vi "Destroy StateMachine.vi"(8 "error in (no error)":errorcluster, 11 "statemachine in":refnum<class "statemachine.lvclass">) -> (0 "error out":errorcluster, 3 "statemachine out":refnum<class "statemachine.lvclass">)   [LabVIEW 2020, in "eos.lvlib" / "statemachine.lvclass"]
uses:
  statemachine.lvclass
  statemachine.lvclass/statemachine.ctl
  interfaces/data/data.lvclass
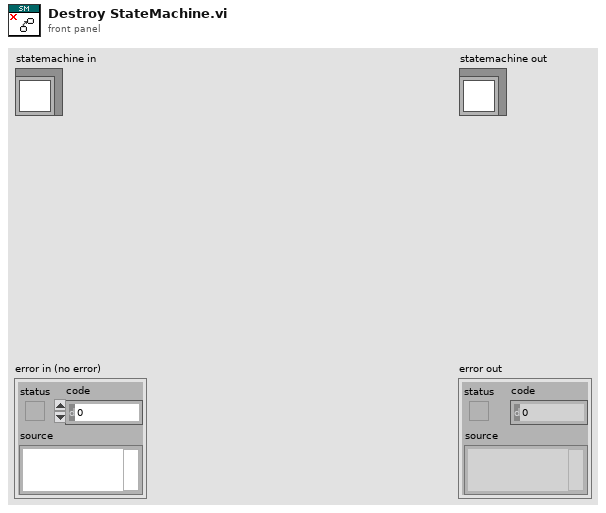
[diagram p1: front panel]
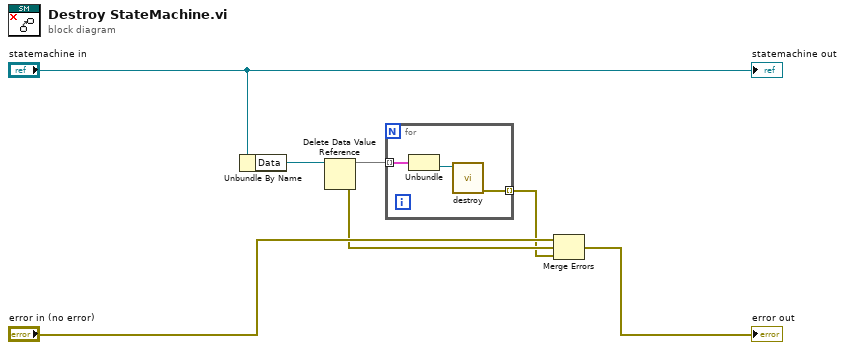
[diagram p0: block diagram]
diagram:
  n1 = Unbundle By Name("statemachine in") -> ("Data"=w4:refnum<data-value>)
  n2 = Delete Data Value Reference(data value reference=w4) -> (data value=w2:map{string, refnum<class "data.lvclass">}, error out=w3:errorcluster)  [unwired: 1 in]
  n3 = for {
    tunnel: w2 -> [w10] mode=indexing
    tunnel: [w8] -> w1 mode=indexing
    n4 = Unbundle(w10) -> ("eos.lvlib:data.lvclass"=w9:refnum<class "data.lvclass">)  [unwired: 1 out]
    n5 = call-dynamic "destroy.vi"("data in"=w9) -> ("error out"=w8:errorcluster)  [unwired: 9 in, 1 out]
  }
  n6 = Merge Errors("error in (no error)", w3, w1) -> (→"error out":errorcluster)
  "statemachine out" <- "statemachine in"
